vi "Wait with Error Clusters.vi"(11 "error in (no error)":errorcluster, 13 "Wait (mS)":u32) -> (15 "error out":errorcluster)   [LabVIEW 2018]
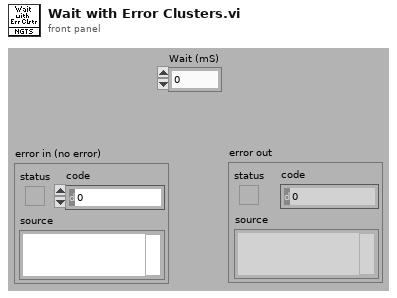
[diagram p1: front panel]
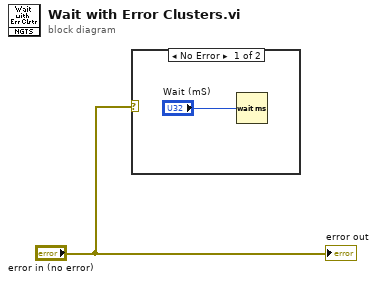
[diagram p0: block diagram]
diagram:
  n1 = case shown="No Error" "error in (no error)" {
    frame No Error {
      n2 = Wait (ms)(milliseconds to wait="Wait (mS)") -> ()  [unwired: 1 out]
    }
    frame Error {
    }
  }
  "error out" <- "error in (no error)"
